vi "Set Virtual Instr Configuration.vi"(8 "error in (no error)":errorcluster, 10 "Virt Instr CFG":string, 11 "IConfiguration UI Actor in":refnum<class "IConfiguration UI Actor.lvclass">) -> (0 "error out":errorcluster, 3 "IConfiguration UI Actor out":refnum<class "IConfiguration UI Actor.lvclass">)   [LabVIEW 2023, in "IConfiguration UI Actor.lvlib" / "IConfiguration UI Actor.lvclass"]
uses:
  IConfiguration UI Actor.lvclass
  <vilib>/ErrorRing/Error Ring.xnode
  <vilib>/Utility/error.llb/Error Cluster From Error Code.vi
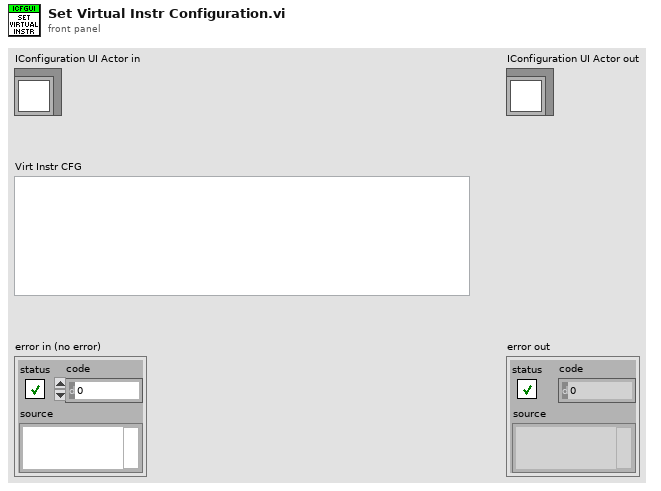
[diagram p1: front panel]
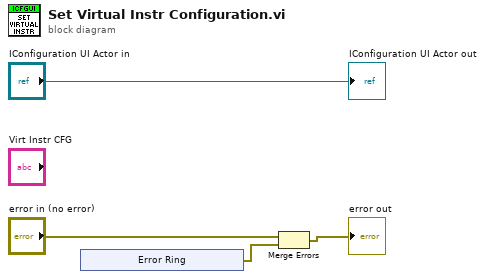
[diagram p0: block diagram]
diagram:
  n1 = xnode "Error Ring"() -> ("error out"=w1:errorcluster)
  n2 = Merge Errors("error in (no error)", w1) -> (→"error out":errorcluster)
  "IConfiguration UI Actor out" <- "IConfiguration UI Actor in"
